vi "merFISH_save_scan_and_prepare next.vi"(3 "List probe Refnum":refnum<vi>, 4 "PATH cluster":T1, 5 "queue CAMERA":refnum<queue>, 6 "queue piezo":refnum<queue>, 7 "error in":errorcluster, 8 "Global parameters":T3={"405"=0.0, "488"=0.0, "561"=0.0, "641"=0.0, "BF"=0.0, "X"=0.0, "Y"=0.0, "Filter list"=1, "Exp time"=0.0, "Kinetic time"=0.0, "Gain"=0, "Step length (nm)"=0, "Total range (nm)"=0, "Scan illumination\n mode"=FALSE, "Dt (s)"=0, "# repetitions"=0} {"# repetitions" min=0; "Dt (s)" min=0 step=1; "Filter list" items=["ET665lp", "zet405/488/561/640m", "None", "None", "None", "None"]}, 9 "ROI list Refnum":refnum<vi>, 10 "Laser list Refnum":refnum<vi>, 11 "Data":T2) -> (0 "error out":errorcluster)   [LabVIEW 2015]
uses:
  CONTROLS/Global parameters.ctl
  CONTROLS/Q_camera_element.ctl
  CONTROLS/Q_MCL_piezo_element.ctl
  GLOBAL/Global_MAIN.vi
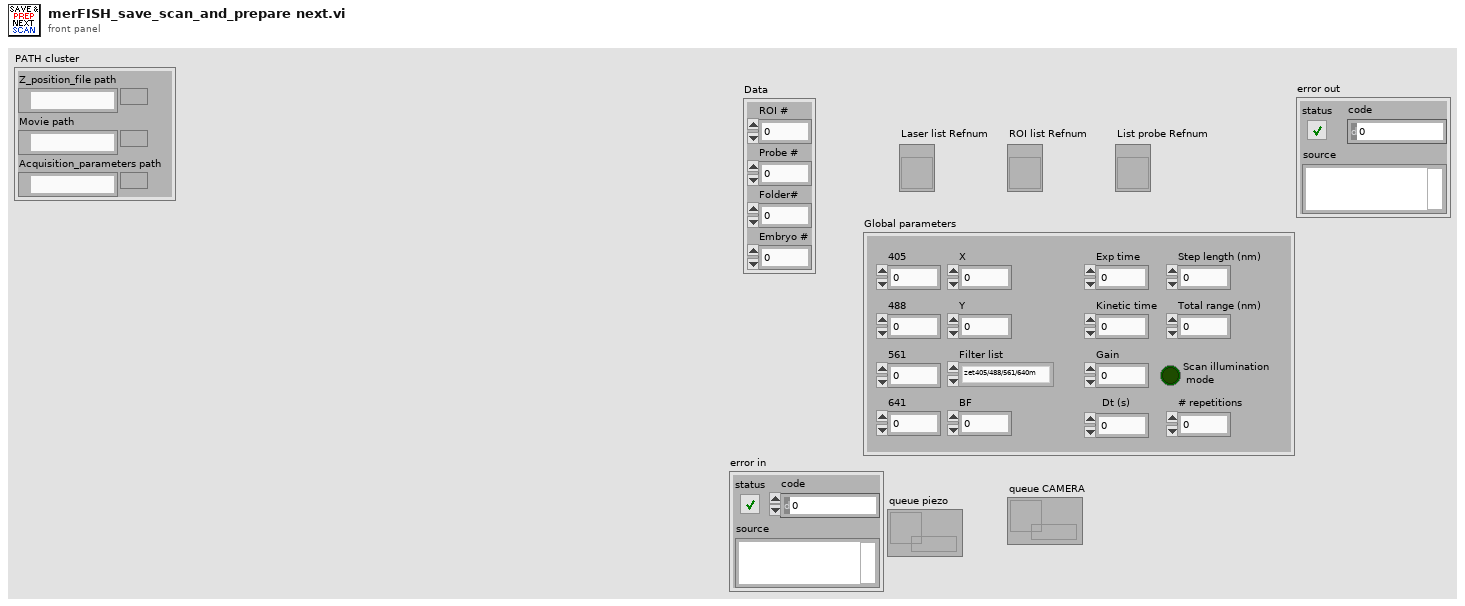
[diagram p1: front panel]
types:
  T1 = cluster{"Z_position_file path":path, "Movie path":path, "Acquisition_parameters path":path}
  T2 = cluster{"ROI #":i32, "Probe #":i32, "Folder# ":i32, "Embryo #":i32}
  T3 = typedef "Global parameters.ctl" = cluster{"405":dbl, "488":dbl, "561":dbl, "641":dbl, "BF":dbl, "X":dbl, "Y":dbl, "Filter list":u16, "Exp time":sgl, "Kinetic time":sgl, "Gain":i32, "Step length (nm)":u32, "Total range (nm)":u32, "Scan illumination\n mode":bool, "Dt (s)":i32, "# repetitions":i32}
  T4 = typedef "Q_camera_element.ctl" = cluster{"variant":variant, "Instruction":enum16{"CAMERA_idle", "CAMERA_initialize", "CAMERA_error", "CAMERA_security_stop", "CAMERA_not_acquiring", "CAMERA_acquiring", "CAMERA_start_acquiring", "CAMERA_stop_acquiring", "CAMERA_change_exposure", "CAMERA_define_ROI", "CAMERA_cooler", "CAMERA_acquire_movie", "CAMERA_init_scan", "CAMERA_check_image_scan", "CAMERA_close_scan", "CAMERA_init_merFISH", "CAMERA_start_acquiring_merFISH", "CAMERA_close_scan_merFISH", "CAMERA_close_merFISH", "CAMERA_STOP"}}
  T5 = typedef "Q_MCL_piezo_element.ctl" = cluster{"variant":variant, "Instruction":enum16{"Piezo_idle", "Piezo_initialize", "Piezo_error", "Piezo_security_stop", "Piezo_read_z", "Piezo_move_z", "Piezo_keyboard_move", "Piezo_close_autofocus_calibration_ramp", "Piezo_change_init_state", "Piezo_init_autofocus", "Piezo_init_autofocus_merFISH_TL", "Piezo_autofocus", "Piezo_autofocus_merFISH_TL", "Piezo_stop_autofocus", "Piezo_stop_autofocus_merFISH_TL", "Piezo_autofocus_lost", "Piezo_resume_autofocus_merFISH_TL", "Piezo_check_z_position_merFISH_TL", "Piezo_init_ramp", "Piezo_move_z_ramp", "Piezo_close_ramp", "Piezo_close_merFISH", "Piezo_stop"}}
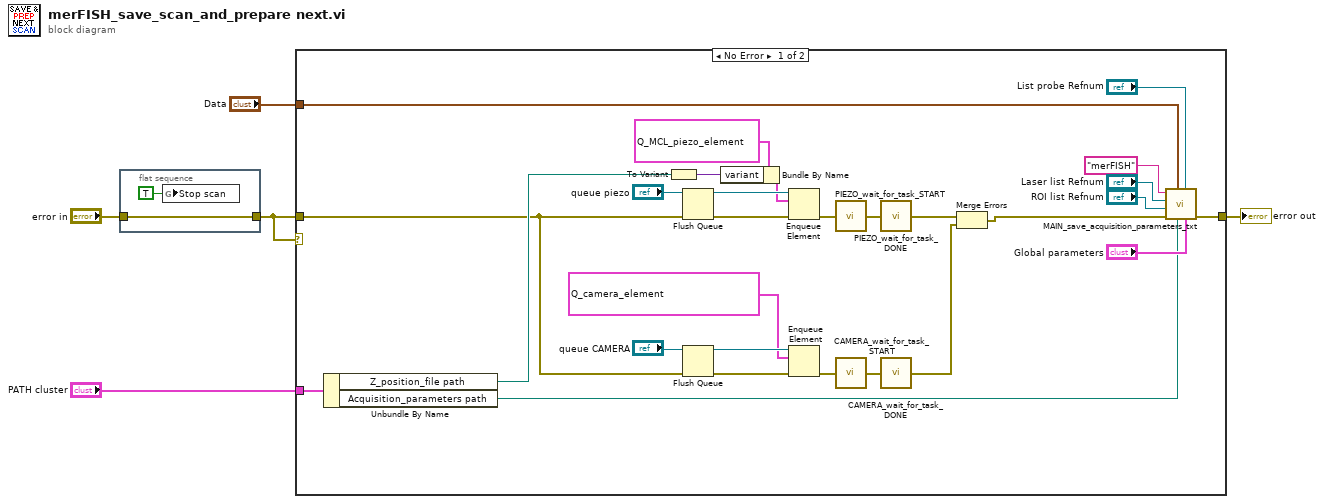
[diagram p0: block diagram]
diagram:
  n1 = flat-sequence {
    tunnel: "error in" -> [w7]
    tunnel: [w7] -> w2
    frame #0 {
      n2 = global write "Global_MAIN.vi" "Stop scan"(TRUE ("Stop scan")) -> ()
    }
  }
  n3 = case shown="No Error" w2 {
    tunnel: w2 -> [w11 w36]
    tunnel: [w12 w36] -> w5
    tunnel: "Data" -> [w17 _]
    tunnel: "PATH cluster" -> [w16 _]
    frame No Error {
      n4 = Unbundle By Name(w16) -> ("Z_position_file path"=w15:path, "Acquisition_parameters path"=w14:path)
      n5 = To Variant(anything=w15) -> (Variant=w33:variant)
      n6 = Flush Queue(queue="queue piezo", error in (no error)=w11) -> (queue out=w32:refnum<queue>, error out=w29:errorcluster)  [unwired: 1 out]
      n7 = Flush Queue(queue="queue CAMERA", error in (no error)=w11) -> (queue out=w26:refnum<queue>, error out=w27:errorcluster)  [unwired: 1 out]
      n8 = Bundle By Name(cluster=T5 {"variant"=variant, "Instruction"=enum."Piezo_close_ramp"} ("Q_MCL_Piezo"), "variant"=w33) -> (w31:T5)
      n9 = Enqueue Element(queue=w32, element=w31, error in (no error)=w29) -> (error out=w34:errorcluster)  [unwired: 1 in, 2 out]
      n10 = Enqueue Element(queue=w26, element=T4 {"variant"=variant, "Instruction"=enum."CAMERA_close_scan_merFISH"} ("Q_ANDOR_element"), error in (no error)=w27) -> (error out=w25:errorcluster)  [unwired: 1 in, 2 out]
      n11 = call "PIEZO_wait_for_task_START.vi"("error in"=w34) -> ("error out"=w35:errorcluster)
      n12 = call "CAMERA_wait_for_task_START.vi"("error in"=w25) -> ("error out"=w24:errorcluster)
      n13 = call "PIEZO_wait_for_task_DONE.vi"("error in"=w35) -> ("error out"=w10:errorcluster)
      n14 = call "CAMERA_wait_for_task_DONE.vi"("error in"=w24) -> ("error out"=w9:errorcluster)
      n15 = Merge Errors(w10, w9) -> (w8:errorcluster)
      n16 = call "MAIN_save_acquisition_parameters_txt.vi"("Global parameters"="Global parameters", "List probe Refnum"="List probe Refnum", "file path"=w14, "Data"=w17, "error in"=w8, "ROI list Refnum"="ROI list Refnum", "Laser list Refnum"="Laser list Refnum", "Data type"="merFISH") -> ("error out"=w12:errorcluster)  [unwired: 3 in]
    }
    frame Error {
    }
  }
  "error out" <- w5
